vi "ClassAttributes_ReadWriteClassAttributes_6x8x6_Singleton.vi"(5 "error in (no error)":errorcluster) -> (19 "error out":errorcluster)   [LabVIEW 2010]
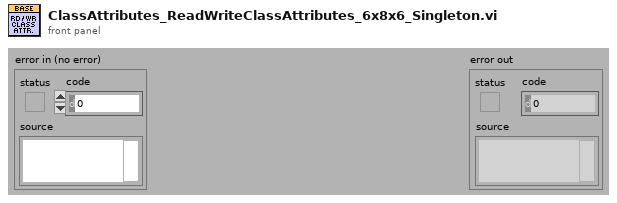
[diagram p1: front panel]
types:
  T1 = typedef "ClassAttributes_ClassAttributes.ctl" = cluster{"classAttribute1":bool}
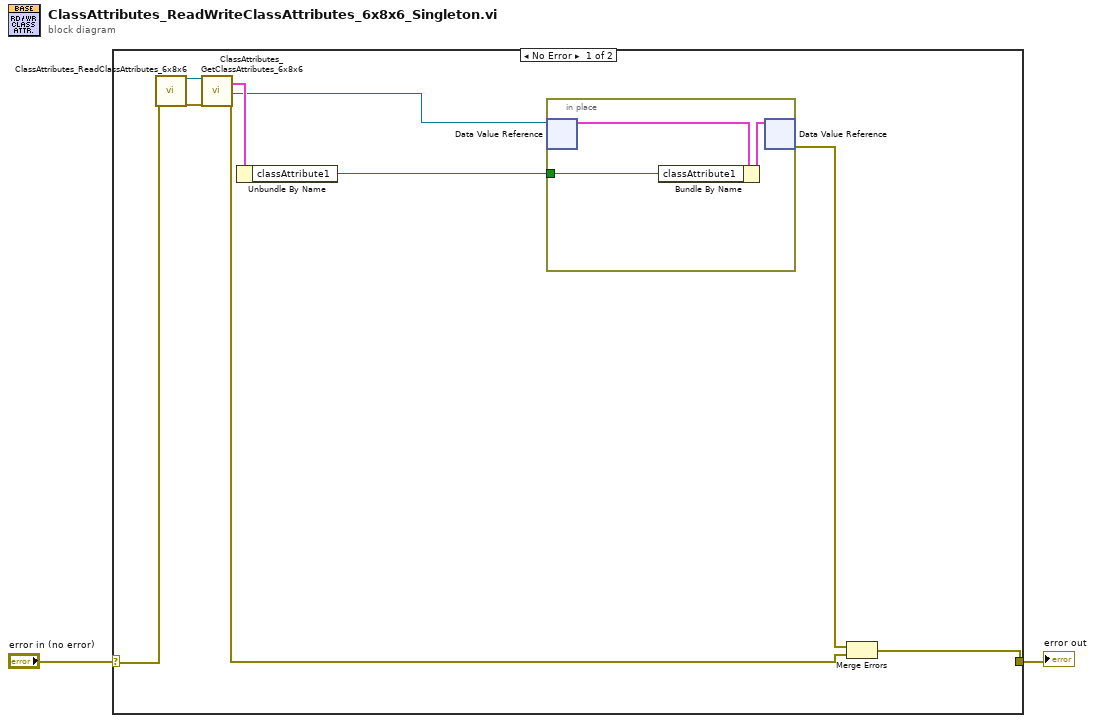
[diagram p0: block diagram]
diagram:
  n1 = case shown="No Error" "error in (no error)" {
    selector: "error in (no error)" -> [w5 w15]
    tunnel: [w8 w15] -> w1
    frame No Error {
      n2 = call "ClassAttributes_ReadClassAttributes_6x8x6.vi"("error in (no error)"=w5) -> ("reference out"=w7:refnum<class>, "error out"=w6:errorcluster)  [unwired: 17 in]
      n3 = call "ClassAttributes_GetClassAttributes_6x8x6.vi"("reference in"=w7, "error in (no error)"=w6) -> ("Class attribute"=w4:T1, "Class attribute Reference"=w3:refnum<data-value>, "error out"=w9:errorcluster)  [unwired: 14 in, 1 out]
      n4 = Unbundle By Name(w4) -> ("classAttribute1"=w10:bool)
      n5 = in-place {
        in-place-border: w10 -> [w14]
        n6 = in-place-dvr #1(w3) -> (w13:T1)  [unwired: 1 out]
        n7 = Bundle By Name(cluster=w13, "classAttribute1"=w14) -> (w12:T1)
        n8 = in-place-dvr #1(w12) -> (w11:errorcluster)  [unwired: 1 out]
      }
      n9 = Merge Errors(w11, w9) -> (w8:errorcluster)
    }
    frame Error {
    }
  }
  "error out" <- w1
